vi "InterfaceNode_Create.vi"(0 "reference":refnum<class "InterfaceNode.lvclass">, 5 "error in (no error)":errorcluster) -> (14 "reference out":refnum<class "InterfaceNode.lvclass">, 19 "error out":errorcluster)   [LabVIEW 2020, in "InterfaceNode.lvclass"]
doc: "Creates and initializes a new InterfaceNode object.\n\nThis object should be destroyed using a InterfaceNode destructor VI or a virtual base class destructor VI.\n\n[GOOP 2.1]"
uses:
  <resource>/Framework/Providers/Open_GDS/UML/InterfaceNode_class/InterfaceNode.lvclass
  C:/Program Files (x86)/National Instruments/LabVIEW 2020/resource/Framework/Providers/Open_GDS/UML/ClassNode_class/ClassNode.lvclass
  <resource>/Framework/Providers/Open_GDS/UML/MultiLineString_class/MultiLineString.lvclass
  <resource>/Framework/Providers/Open_GDS/UML/ClassNode_class/ClassNode.lvclass
panel:
  # "The input reference should only\nbe wired when this method is called\nby a sub class constructor."
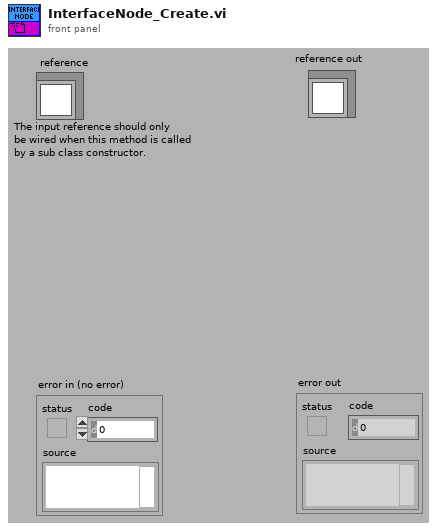
[diagram p1: front panel]
types:
  T1 = typedef "InterfaceNode.lvclass/ObjectAttributes.ctl" = cluster{"None":bool}
  T2 = typedef "ClassNode.lvclass/ObjectAttributes.ctl" = cluster{"midHeight":dbl, "botHeight":dbl, "name":refnum<class "MultiLineString.lvclass">, "attributes":refnum<class "MultiLineString.lvclass">, "methods":refnum<class "MultiLineString.lvclass">, "DEFAULT_COMPARTMENT_HEIGHT":i32, "DEFAULT_WIDTH":i32, "DEFAULT_HEIGHT":i32, "showMethods":bool, "showAttributes":bool, "ClassPath":path}
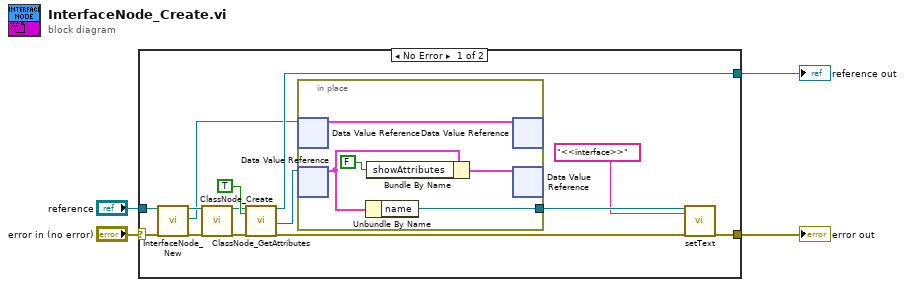
[diagram p0: block diagram]
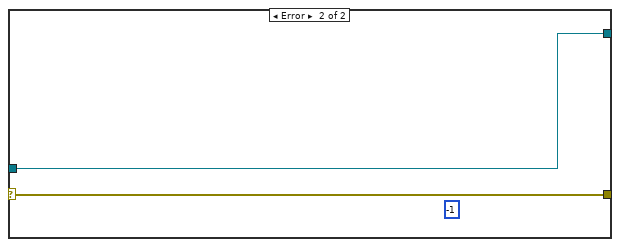
[diagram p2: hidden frame]
diagram:
  n1 = case shown="No Error" "error in (no error)" {
    selector: "error in (no error)" -> [w18 w25]
    tunnel: [w14 w24] -> w4
    tunnel: [w6 w25] -> w3
    tunnel: "reference" -> [w17 w24]
    frame No Error {
      n2 = call <resource>:"InterfaceNode_New.vi"("reference in"=w17, "error in (no error)"=w18) -> ("reference out"=w15:refnum<class "InterfaceNode.lvclass">, "DVRRefOut"=w11:refnum<data-value>, "error out"=w16:errorcluster)  [unwired: 2 in, 13 out]
      n3 = call <resource>:"ClassNode_Create.vi"("reference"=w15, "error in (no error)"=w16) -> ("reference out"=w9:refnum<class "InterfaceNode.lvclass">, "error out"=w10:errorcluster)  [unwired: 16 in]
      n4 = call <resource>:"ClassNode_GetAttributes.vi"("reference in"=w9, "OnlyGetDvrReference(False)"=TRUE, "error in (no error)"=w10) -> ("reference out"=w14:refnum<class "InterfaceNode.lvclass">, "DataRef"=w12:refnum<data-value>, "error out"=w7:errorcluster)  [unwired: 13 in, 1 out]
      n5 = in-place {
        in-place-border: [w19] -> w8
        n6 = in-place-dvr #1(w11) -> (w22:T1)  [unwired: 1 out]
        n7 = in-place-dvr #2(w12) -> (w20:T2)  [unwired: 1 out]
        n8 = Unbundle By Name(w20) -> ("name"=w19:refnum<class "MultiLineString.lvclass">)
        n9 = Bundle By Name(cluster=w20, "showAttributes"=FALSE) -> (w23:T2)
        n10 = in-place-dvr #1(w22) -> ()  [unwired: 2 out]
        n11 = in-place-dvr #2(w23) -> ()  [unwired: 2 out]
      }
      n12 = call-dynamic "setText.vi"("reference"=w8, "text"="<<interface>>", "error in (no error)"=w7) -> ("error out"=w6:errorcluster)  [unwired: 15 in, 1 out]
    }
    frame Error {
      (unwired) -1 ("Nr of open handles")
    }
  }
  "error out" <- w3
  "reference out" <- w4
